vi "SPI Main.vi"   [LabVIEW 2018]
uses:
  <vilib>/eio/EIONode/EIONode.xnode
  <vilib>/rvi/eio/common/nirviEmuTemplateMethod_errors.vi
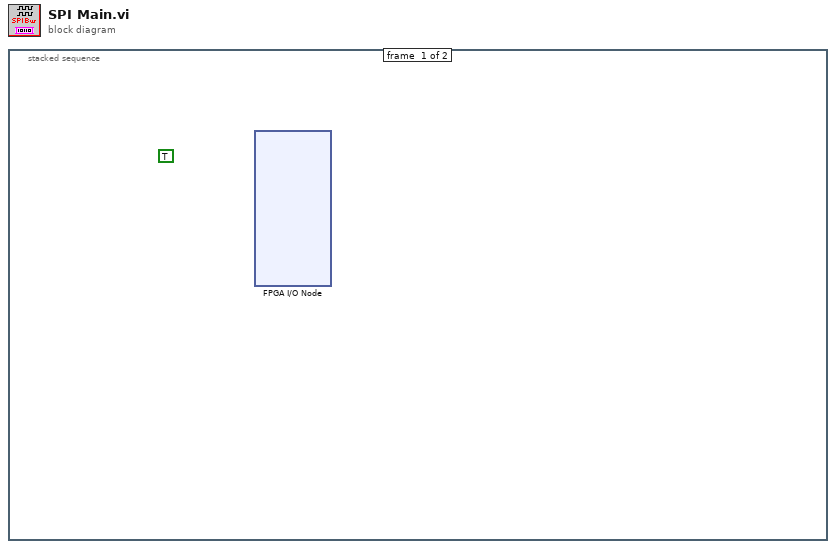
[diagram p0: block diagram]
diagram:
  n1 = stacked-sequence {
    frame #0 {
      (unwired) TRUE
      n2 = xnode "FPGA I/O Node"() -> ()  [unwired: 16 in, 8 out]
    }
    frame #1 {
    }
  }
